vi "Z-Scan-offset-ref.vi"(1 "Array in":dbl[](array[numeric])) -> (0 "Array out":dbl[](array[numeric]))   [LabVIEW 2014]
doc: "Andre Romero - 2016\nandretec@ifsc.usp.br"
panel:
  out "Waveform Graph 2":dbl[](graph)
  out "Waveform Graph":dbl[](graph)
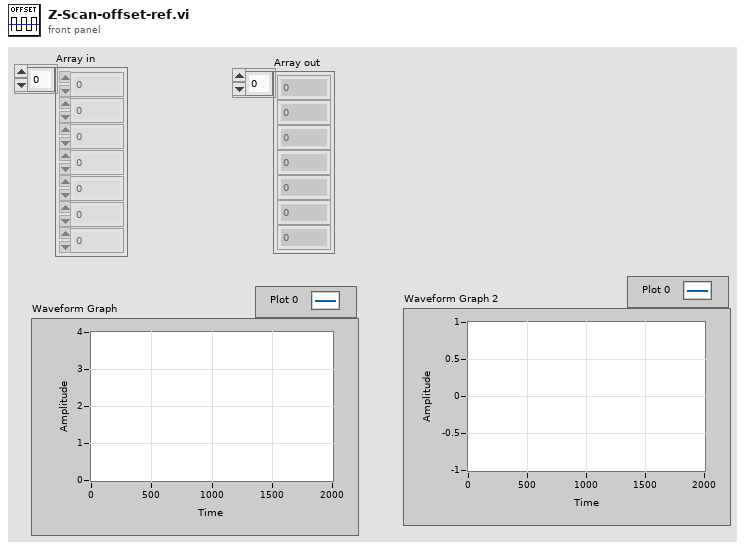
[diagram p1: front panel]
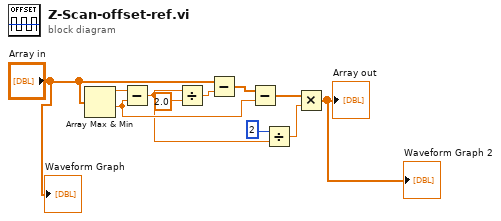
[diagram p0: block diagram]
diagram:
  n1 = Array Max & Min(array="Array in") -> (max value=w9:dbl, min value=w7:dbl)  [unwired: 2 out]
  n2 = Subtract(x=w9, y=w7) -> (x-y=w4:dbl)
  n3 = Divide(x=w4, y=2.0) -> (x/y=w11:dbl)
  n4 = Subtract(x="Array in", y=w11) -> (x-y=w8:dbl[])
  n5 = Subtract(x=w8, y=w7) -> (x-y=w6:dbl[])
  n6 = Divide(x=2, y=w4) -> (x/y=w3:dbl)
  n7 = Multiply(x=w6, y=w3) -> (x*y=→"Array out" →"Waveform Graph 2":dbl[])
  "Waveform Graph" <- "Array in"
